vi "1.1.vi"() -> ()   [LabVIEW 2017]
panel:
  in  "停止":bool
  in  "随机数生产":bool
  out "随机数":dbl
  in  "?":sgl=5.0 min=0 max=10 step=0.1
  out "显示结果":bool
  # "比较数字"
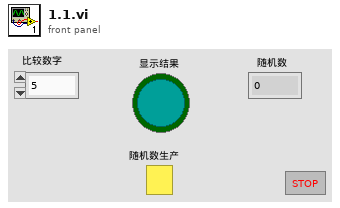
[diagram p1: front panel]
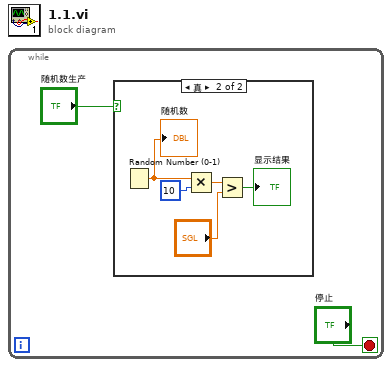
[diagram p0: block diagram]
diagram:
  n1 = while {
    stop <- "停止" stop-if-true
    n2 = case shown="真" "随机数生产" {
      frame False {
      }
      frame True {
        n3 = Random Number (0-1)() -> (number: 0 to 1=w7:dbl)
        "随机数" <- w7
        n4 = Multiply(x=w7, y=10) -> (x*y=w5:dbl)
        n5 = Greater?(x=w5, y="?") -> (0:→"显示结果":bool)
      }
    }
  }
